vi "GV-CursorVzoom.vi"(6 "Y":dbl, 7 "Gviewer in":refnum<class "Gviewer.lvclass">, 8 "error in (no error)":errorcluster, 10 "Pos":cluster{"x":i16, "y":i16}, 11 "pict in":picture) -> (0 "error out":errorcluster, 3 "pict out":picture)   [LabVIEW 2020, in "Gviewer.lvclass"]
doc: "Andre Koelewijn, 30 jan 2021\n\nVertical scroll zoom cursor draw"
uses:
  Gviewer.lvclass
  Gviewer.lvclass/Gviewer.ctl
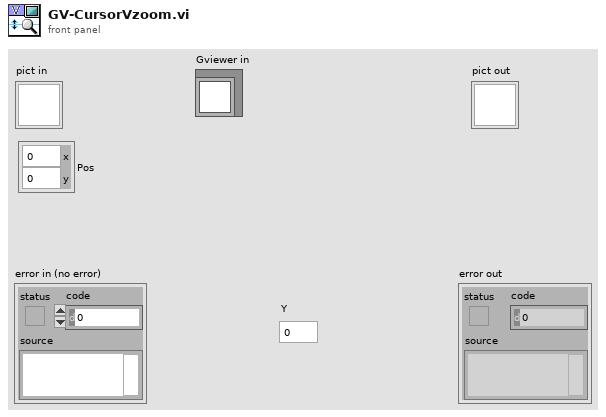
[diagram p1: front panel]
types:
  T1 = cluster{"horizontal":enum16{"left", "center", "right"}, "vertical":enum16{"top", "center", "bottom"}}
  T2 = cluster{"Width":u16, "Style":enum32{"Solid", "Dash", "Dot", "DashDot", "DashDotDot"}}
  T3 = typedef "Gviewer.lvclass/Typedef_SelProperties.ctl" = cluster{"Color":u32, "LineType":T4, "max":dbl, "min":dbl}
  T4 = typedef "Gviewer.lvclass/Typedef_LineType.ctl" = enum16{"num_bare", "num_MinMax_Area", "num_MinMax_Lines", "num_MinMax_Forfor", "num_Max_Area", "num_Max_Line", "num_Max_Forfor", "num_Min_Area", "num_Min_Line", "num_Min_Fosfor", "Boolean_Line_01", "Boolean_Area_01", "Boolean_Fosfor_01", "Boolean_Line_TF", "Boolean_Area_TF", "Boolean_Fosfor_TF", "Boolean_OnOff_Line", "Boolean_OnOff_Area", "Boolean_OnOff_Fosfor", "Boolean_spare", "StringEvent_Line", "StringEvent_TimeLine"}
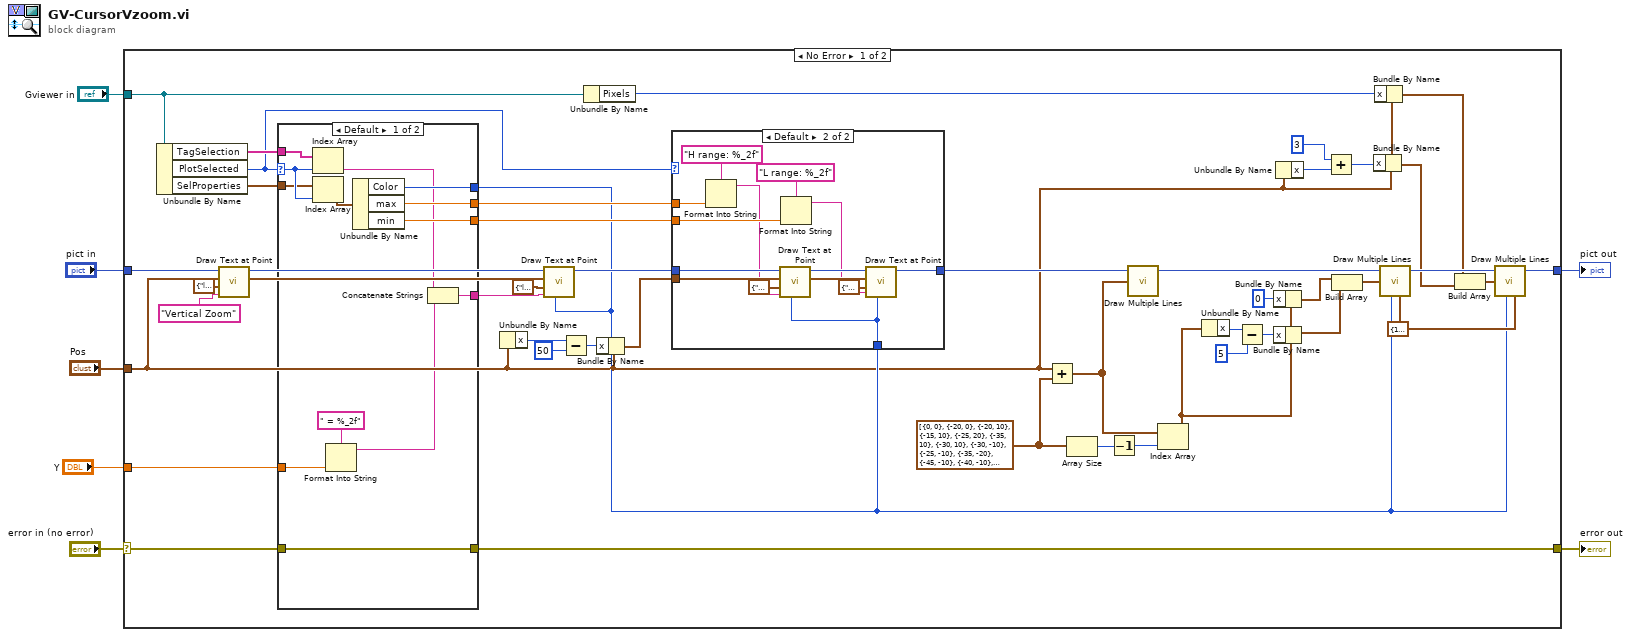
[diagram p0: block diagram]
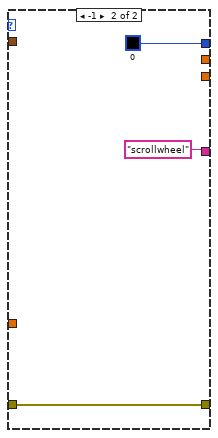
[diagram p3: hidden frame]
diagram:
  n1 = case shown="No Error" "error in (no error)" {
    selector: "error in (no error)" -> [w12 w85]
    tunnel: [w11 w85] -> w6
    tunnel: "pict in" -> [w29 w84]
    tunnel: [w38 w84] -> w4
    tunnel: "Pos" -> [w10 _]
    tunnel: "Gviewer in" -> [w23 _]
    tunnel: "Y" -> [w8 _]
    frame No Error {
      w47 = T2 {"Width"=1, "Style"=enum."Dash"} ("pen")
      w52 = cluster{"x":i16, "y":i16}[] [{"x"=0, "y"=0}, {"x"=-20, "y"=0}, {"x"=-20, "y"=10}, {"x"=-15, "y"=10}, {"x"=-25, "y"=20}, {"x"=-35, "y"=10}, {"x"=-30, "y"=10}, {"x"=-30, "y"=-10}, {"x"=-25, "y"=-10}, {"x"=-35, "y"=-20}, {"x"=-45, "y"=-10}, {"x"=-40, "y"=-10}, {"x"=-40, "y"=0}, {"x"=-50, "y"=0}] ("line endpoints")
      n2 = Unbundle By Name(w23) -> ("TagSelection"=w26:string[], "PlotSelected"=w9:i32, "SelProperties"=w28:T3[])
      n3 = call <vilib>:"Draw Text at Point.vi"("text"="Vertical Zoom", "alignment(left, top)"=T1 {"horizontal"=enum."left", "vertical"=enum."bottom"}, "origin"=w10, "picture"=w29) -> ("new picture"=w24:picture)  [unwired: 6 in, 1 out]
      n4 = case shown="Default" w9 {
        selector: w9 -> [w77 _]
        tunnel: w26 -> [w80 _]
        tunnel: [w73 "scrollwheel"] -> w27
        tunnel: w28 -> [w72 _]
        tunnel: [w78 u32 0 ("Color")] -> w13
        tunnel: [w76 _] -> w20
        tunnel: [w75 _] -> w19
        tunnel: w12 -> [w69 w81]
        tunnel: [w69 w81] -> w11
        tunnel: w8 -> [w68 _]
        frame Default {
          n5 = Index Array(array=w80, index=w77) -> (element=w74:string)
          n6 = Index Array(array=w72, index=w77) -> (element=w79:T3)
          n7 = Format Into String(format string=" = %_2f", w68) -> (resulting string=w70:string)  [unwired: 2 in, 1 out]
          n8 = Unbundle By Name(w79) -> ("Color"=w78:u32, "max"=w76:dbl, "min"=w75:dbl)
          n9 = Concatenate Strings(w74, w70) -> (w73:string)
        }
        frame -1 {
        }
      }
      n10 = Unbundle By Name(w10) -> ("x"=w17:i16)
      n11 = call <vilib>:"Draw Text at Point.vi"("text color(black)"=w13, "text"=w27, "alignment(left, top)"=T1 {"horizontal"=enum."left", "vertical"=enum."top"}, "origin"=w10, "picture"=w24) -> ("new picture"=w21:picture)  [unwired: 5 in, 1 out]
      n12 = Subtract(x=w17, y=i16 50) -> (x-y=w15:i16)
      n13 = Unbundle By Name(w23) -> ("Pixels"=w22:i32)
      n14 = Bundle By Name(cluster=w10, "x"=w15) -> (w14:cluster{"x":i16, "y":i16})
      n15 = case shown="Default" w9 {
        tunnel: w21 -> [w54 w66]
        tunnel: w20 -> [_ w62]
        tunnel: w19 -> [_ w61]
        tunnel: [w54 w63] -> w18
        tunnel: w14 -> [_ w60]
        tunnel: w13 -> [_ w55]
        frame -1 {
        }
        frame Default {
          n16 = Format Into String(format string="H range: %_2f", w62) -> (resulting string=w56:string)  [unwired: 2 in, 1 out]
          n17 = call <vilib>:"Draw Text at Point.vi"("text color(black)"=w55, "text"=w56, "alignment(left, top)"=T1 {"horizontal"=enum."right", "vertical"=enum."bottom"}, "origin"=w60, "picture"=w66) -> ("new picture"=w64:picture)  [unwired: 5 in, 1 out]
          n18 = Format Into String(format string="L range: %_2f", w61) -> (resulting string=w57:string)  [unwired: 2 in, 1 out]
          n19 = call <vilib>:"Draw Text at Point.vi"("text color(black)"=w55, "text"=w57, "alignment(left, top)"=T1 {"horizontal"=enum."right", "vertical"=enum."top"}, "origin"=w60, "picture"=w64) -> ("new picture"=w63:picture)  [unwired: 5 in, 1 out]
        }
      }
      n20 = Add(x=w10, y=w52) -> (x+y=w49:cluster{"x":i16, "y":i16}[])
      n21 = Array Size(array=w52) -> (size(s)=w51:i32)
      n22 = Decrement(x=w51) -> (x-1=w50:i32)
      n23 = call <vilib>:"Draw Multiple Lines.vi"("picture"=w18, "line endpoints"=w49) -> ("new picture"=w53:picture)  [unwired: 7 in]
      n24 = Index Array(array=w49, index=w50) -> (element=w41:cluster{"x":i16, "y":i16})
      n25 = Unbundle By Name(w41) -> ("x"=w46:i16)
      n26 = Subtract(x=w46, y=i16 5) -> (x-y=w44:i16)
      n27 = Bundle By Name(cluster=w41, "x"=i16 0) -> (w40:cluster{"x":i16, "y":i16})
      n28 = Bundle By Name(cluster=w41, "x"=w44) -> (w43:cluster{"x":i16, "y":i16})
      n29 = Unbundle By Name(w10) -> ("x"=w37:i16)
      n30 = Add(x=i16 3, y=w37) -> (x+y=w36:i16)
      n31 = Build Array(w40, w43) -> (w48:cluster{"x":i16, "y":i16}[])
      n32 = Bundle By Name(cluster=w10, "x"=w36) -> (w33:cluster{"x":i16, "y":i16})
      n33 = Bundle By Name(cluster=w10, "x"=w22) -> (w32:cluster{"x":i16, "y":i16})
      n34 = call <vilib>:"Draw Multiple Lines.vi"("picture"=w53, "line endpoints"=w48, "color(black)"=w13, "pen"=w47) -> ("new picture"=w39:picture)  [unwired: 5 in]
      n35 = Build Array(w32, w33) -> (w34:cluster{"x":i16, "y":i16}[])
      n36 = call <vilib>:"Draw Multiple Lines.vi"("picture"=w39, "line endpoints"=w34, "color(black)"=w13, "pen"=w47) -> ("new picture"=w38:picture)  [unwired: 5 in]
    }
    frame Error {
    }
  }
  "error out" <- w6
  "pict out" <- w4
